vi "Volume of Cylinder.vi"() -> ()   [LabVIEW 2011]
panel:
  out "Volume":dbl(knob) scale=0.0..50.0
  in  "Height":dbl(knob) scale=0.0..10.0
  in  "Radius":dbl(slide) scale=0.0..10.0
  in  "Stop":bool
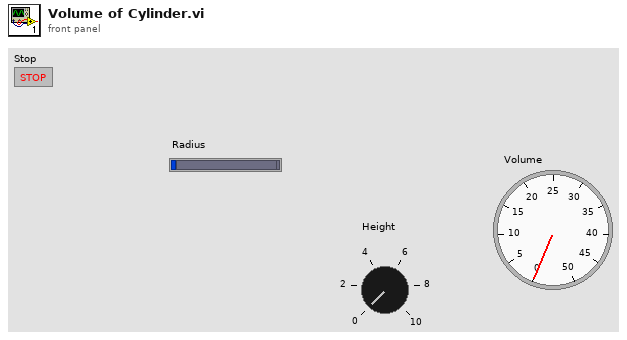
[diagram p1: front panel]
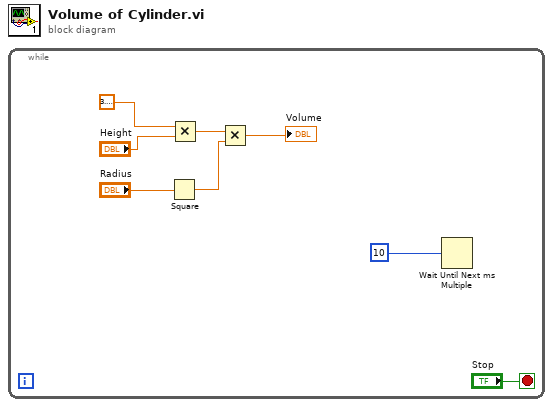
[diagram p0: block diagram]
diagram:
  n1 = while {
    stop <- "Stop" stop-if-true
    n2 = Square(x="Radius") -> (x^2=w4:dbl)
    n3 = Multiply(x=3.141592653589793, y="Height") -> (x*y=w3:dbl)
    n4 = Multiply(x=w3, y=w4) -> (x*y=→"Volume":dbl)
    n5 = Wait Until Next ms Multiple(millisecond multiple=u32 10 ("millisecond timer value")) -> ()  [unwired: 1 out]
  }
